vi "DSF.Engine.Pointer.DBL.Set Channel Count.vi"(10 "channel count":u64, 11 "DBL Buffer in":refnum<class "DSF.Engine.Pointer.DBL.lvclass">) -> (3 "DBL Buffer out":refnum<class "DSF.Engine.Pointer.DBL.lvclass">)   [LabVIEW 2017, in "DSF.Engine.lvlib" / "DSF.Engine.Pointer.DBL.lvclass"]
uses:
  DSF.Engine.Pointer.DBL.lvclass
  DSF.Engine.Pointer.DBL.lvclass/DSF.Engine.Pointer.DBL.ctl
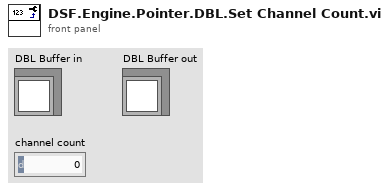
[diagram p1: front panel]
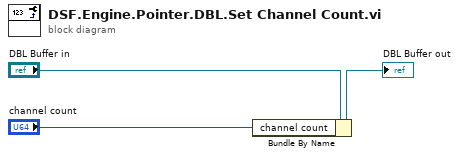
[diagram p0: block diagram]
diagram:
  n1 = Bundle By Name(cluster="DBL Buffer in", "channel count"="channel count") -> (→"DBL Buffer out":refnum<class "DSF.Engine.Pointer.DBL.lvclass">)
